vi "Read DAQ.vi"(8 "error in (no error)":errorcluster, 11 "eCRDS in":refnum<class "eCRDS.lvclass">) -> (0 "error out":errorcluster, 2 "DAQ":T1={"Rate (MHz)"=4.0, "Laser Rep (Hz)"=2000.0, "Laser DC (%)"=0.5}, 3 "eCRDS out":refnum<class "eCRDS.lvclass">)   [LabVIEW 2014, in "eCRDS Library.lvlib" / "eCRDS.lvclass"]
uses:
  eCRDS.lvclass
  eCRDS.lvclass/eCRDS.ctl
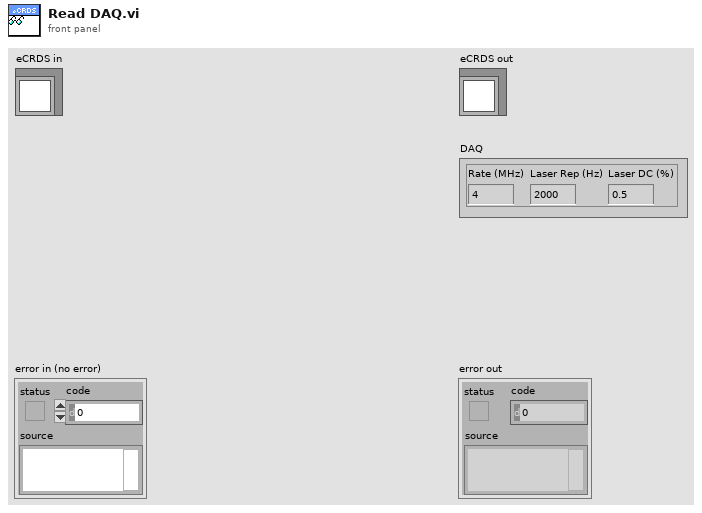
[diagram p1: front panel]
types:
  T1 = cluster{"Rate (MHz)":dbl, "Laser Rep (Hz)":dbl, "Laser DC (%)":dbl}
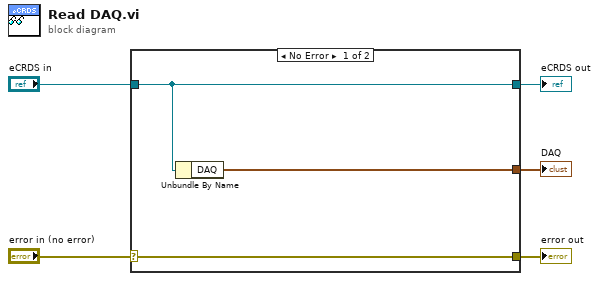
[diagram p0: block diagram]
diagram:
  n1 = case shown="No Error" "error in (no error)" {
    selector: "error in (no error)" -> [w8 w9]
    tunnel: [w8 w9] -> w4
    tunnel: [w7 w10] -> w2
    tunnel: "eCRDS in" -> [w7 w10]
    tunnel: [w6 _] -> w1
    frame No Error {
      n2 = Unbundle By Name(w7) -> ("DAQ"=w6:T1)
    }
    frame Error {
    }
  }
  "error out" <- w4
  "eCRDS out" <- w2
  "DAQ" <- w1
